vi "some type random.vi"() -> ()   [LabVIEW 2018, in "LV2Julia_core.lvlib"]
uses:
  LV2Julia_core.lvlib
  dd189859-e5ca-475d-ae95-e566ebf0657e.vi
  rnd(span).vi
panel:
  out "Numeric out":u64
  in  "Numeric":u64
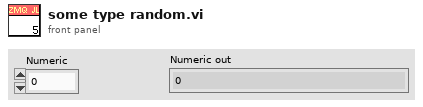
[diagram p1: front panel]
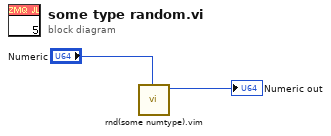
[diagram p0: block diagram]
diagram:
  n1 = call "rnd(some numtype).vim"("type"="Numeric") -> ("Numeric out"=→"Numeric out":u64)  [unwired: 10 in]
